vi "S read array.vi"(11 "array str":string="%f") -> (3 "array":dbl[][](array[numeric]))   [LabVIEW 2010]
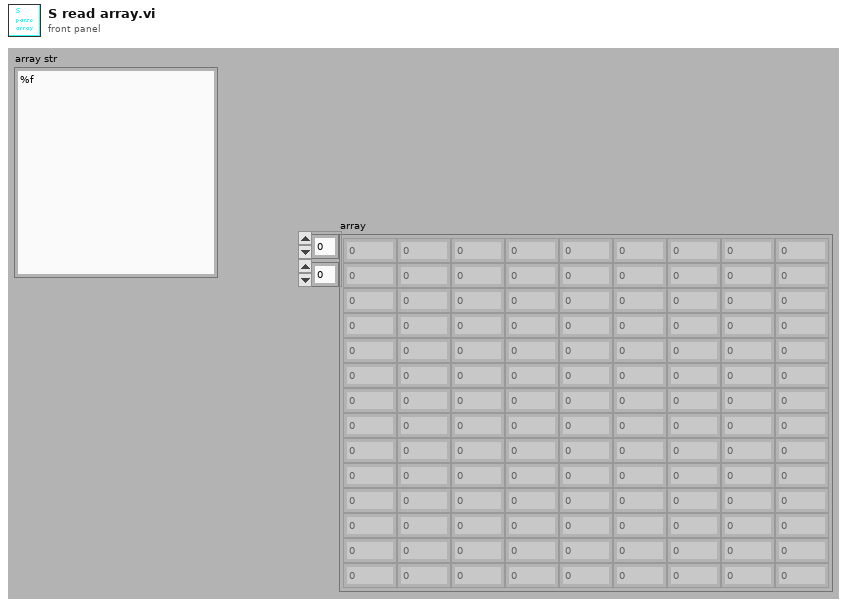
[diagram p1: front panel]
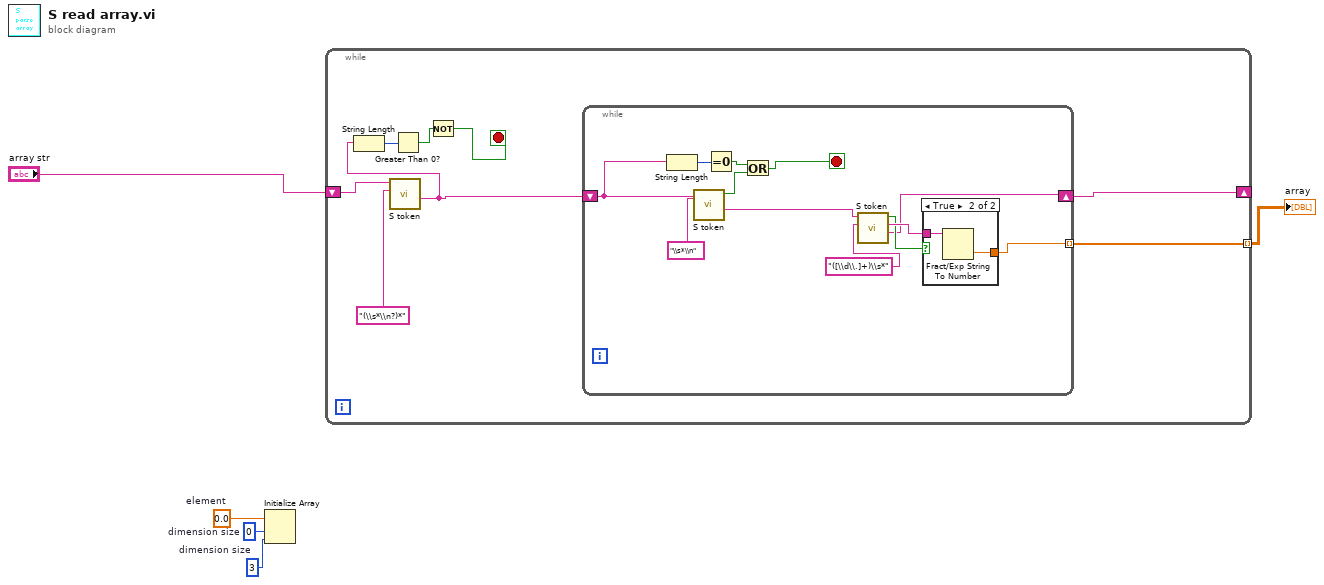
[diagram p0: block diagram]
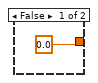
[diagram p2: hidden frame]
diagram:
  w2 = 3  # dimension size
  w3 = 0  # dimension size
  w4 = 0.0  # element
  n1 = Initialize Array(w4, w3, w2) -> ()  [unwired: 1 out]
  n2 = while {
    shift-right: [w13] -> _
    shift-left: "array str" -> [w11]
    tunnel: [w9] -> w1 mode=indexing
    stop <- w6 stop-if-true
    n3 = call "S token.vi"("regular expression"="(\\s*\\n?)*" ("action"), "input string"=w11) -> ("after match"=w8:string)  [unwired: 7 in, 2 out]
    n4 = String Length(string=w8) -> (length=w12:i32)
    n5 = Greater Than 0?(x=w12) -> (x > 0?=w7:bool)
    n6 = Not(x=w7) -> (.not. x?=w6:bool)
    n7 = while {
      shift-right: [w15] -> w13
      shift-left: w8 -> [w18]
      tunnel: [w25] -> w9 mode=indexing
      stop <- w14 stop-if-true
      n8 = String Length(string=w18) -> (length=w24:i32)
      n9 = call "S token.vi"("regular expression"="\\s*\\n" ("action"), "input string"=w18) -> ("after match"=w17:string, "token found"=w19:bool)  [unwired: 7 in, 1 out]
      n10 = Equal To 0?(x=w24) -> (x = 0?=w23:bool)
      n11 = Or(x=w23, y=w19) -> (x .or. y?=w14:bool)
      n12 = call "S token.vi"("regular expression"="([\\d\\.]+)\\s*" ("action"), "input string"=w17) -> ("after match"=w15:string, "whole match"=w21:string, "token found"=w16:bool)  [unwired: 7 in]
      n13 = case shown="True" w16 {
        tunnel: [0.0 w28] -> w25
        tunnel: w21 -> [_ w27]
        frame False {
        }
        frame True {
          n14 = Fract/Exp String To Number(string=w27) -> (number=w28:dbl)  [unwired: 3 in, 1 out]
        }
      }
    }
  }
  "array" <- w1
